vi "Emballage_BDD_bdd_config_emb_Verif.vi"(8 "Error in":errorcluster caption="Error in (no error)", 11 "tableau_config":string[](array[string])) -> (0 "Error out":errorcluster)   [LabVIEW 2020]
uses:
  Modules/Fonction Standard/Email/InfoEmail.ctl
  Modules/FS/60_FS_Controles/60_FS_SetGet.ctl
panel:
  in  "Nom_table":string="Emballage"
  out "resulting string":string
  out "deltaTime [ms]":u32
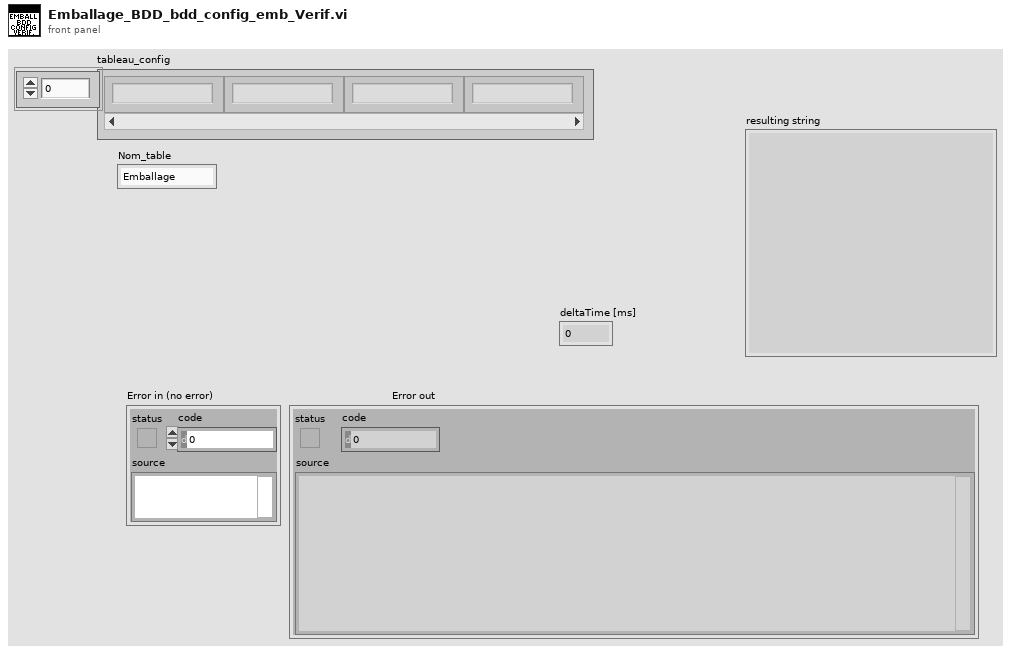
[diagram p1: front panel]
types:
  T1 = typedef "InfoEmail.ctl" = cluster{"Expediteur":string, "Destinataires":string[], "Sujet":string, "Fichier":string, "Message":string}
  T2 = typedef "60_FS_SetGet.ctl" = enum16{"set", "get"}
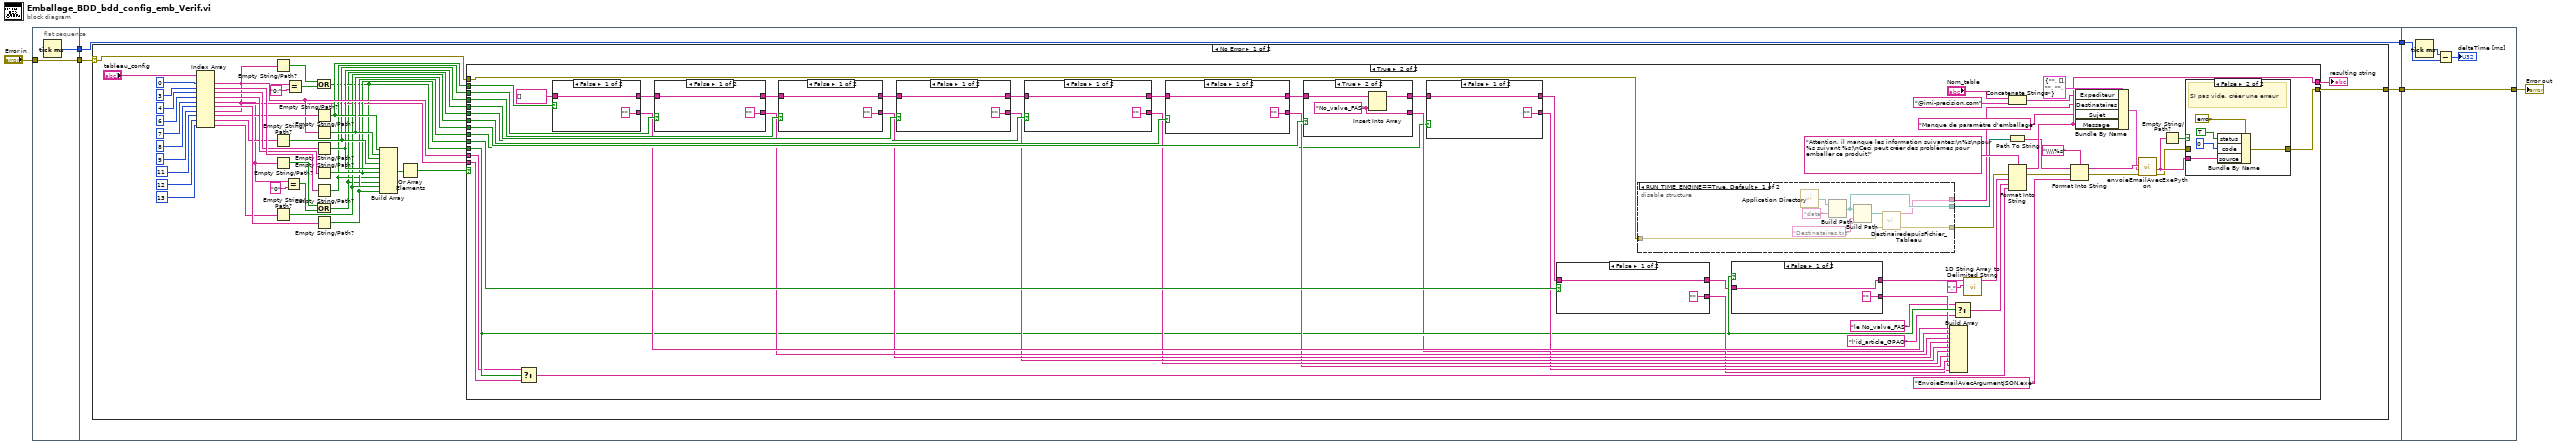
[diagram p0: block diagram]
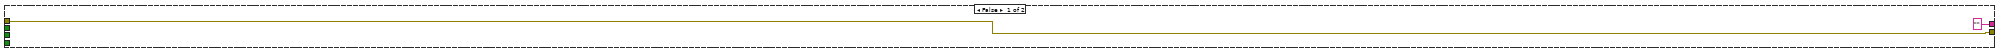
[diagram p2: hidden frame]
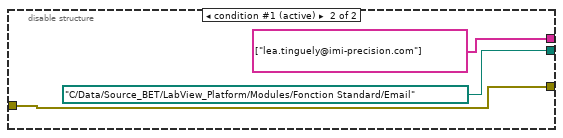
[diagram p3: hidden frame]
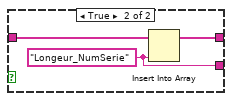
[diagram p5: hidden frame]
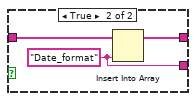
[diagram p6: hidden frame]
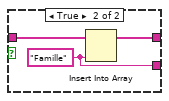
[diagram p7: hidden frame]
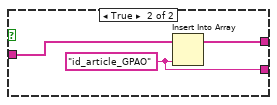
[diagram p8: hidden frame]
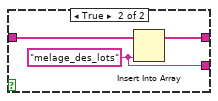
[diagram p9: hidden frame]
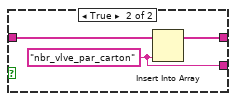
[diagram p10: hidden frame]
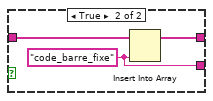
[diagram p11: hidden frame]
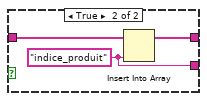
[diagram p12: hidden frame]
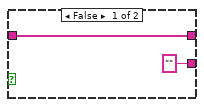
[diagram p13: hidden frame]
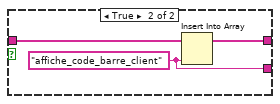
[diagram p14: hidden frame]
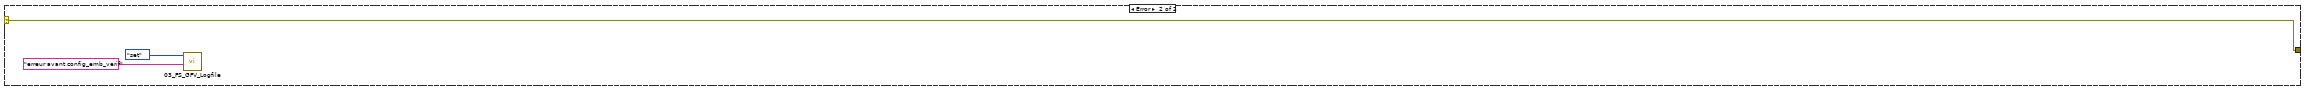
[diagram p15: hidden frame]
diagram:
  n1 = flat-sequence {
    tunnel: "Error in" -> [w8]
    tunnel: [w8] -> w3
    tunnel: [w7] -> w2
    tunnel: [w10] -> w4
    tunnel: w3 -> [w11]
    tunnel: w2 -> [w9]
    tunnel: [w9] -> w1
    tunnel: [w190] -> w5
    tunnel: w4 -> [w190]
    tunnel: w1 -> [w188]
    frame #0 {
      n2 = Tick Count (ms)() -> (millisecond timer value=w7:u32)
    }
    frame #1 {
      n3 = case shown="No Error" w11 {
        selector: w11 -> [w33 w186]
        tunnel: [w34 w186] -> w10
        frame No Error {
          n4 = Index Array(array="tableau_config", index #1=0 ("index"), index #2=3 ("index"), index #3=4 ("index"), index #4=6 ("index"), index #5=7 ("index"), index #6=8 ("index"), index #7=9 ("index"), index #8=11 ("index"), index #9=12 ("index"), index #10=13 ("index")) -> (element #1=w35:string, element #2=w42:string, element #3=w41:string, element #4=w40:string, element #5=w15:string, element #6=w39:string, element #7=w20:string, element #8=w38:string, element #9=w37:string, element #10=w36:string)
          n5 = Empty String/Path?(string/path=w20) -> (empty?=w23:bool)
          n6 = Empty String/Path?(string/path=w37) -> (empty?=w29:bool)
          n7 = Empty String/Path?(string/path=w15) -> (empty?=w13:bool)
          n8 = Empty String/Path?(string/path=w36) -> (empty?=w25:bool)
          n9 = Equal?(x=w15, y="0") -> (x = y?=w12:bool)
          n10 = Equal?(x=w20, y="0;") -> (x = y?=w17:bool)
          n11 = Or(x=w23, y=w17) -> (x .or. y?=w18:bool)
          n12 = Empty String/Path?(string/path=w38) -> (empty?=w30:bool)
          n13 = Empty String/Path?(string/path=w35) -> (empty?=w31:bool)
          n14 = Empty String/Path?(string/path=w41) -> (empty?=w28:bool)
          n15 = Empty String/Path?(string/path=w40) -> (empty?=w27:bool)
          n16 = Empty String/Path?(string/path=w42) -> (empty?=w21:bool)
          n17 = Or(x=w13, y=w12) -> (x .or. y?=w14:bool)
          n18 = Empty String/Path?(string/path=w39) -> (empty?=w24:bool)
          n19 = Build Array(w30, w31, w18, w29, w28, w27, w21, w14, w25, w24) -> (w22:bool[])
          n20 = Or Array Elements(Boolean array=w22) -> (logical OR=w26:bool)
          n21 = case shown="True" w26 {
            tunnel: w31 -> [_ w116]
            tunnel: w21 -> [_ w115]
            tunnel: w28 -> [_ w114]
            tunnel: w27 -> [_ w113]
            tunnel: w14 -> [_ w112]
            tunnel: w24 -> [_ w90]
            tunnel: w30 -> [_ w111]
            tunnel: w29 -> [_ w110]
            tunnel: w25 -> [_ w109]
            tunnel: w18 -> [_ w95]
            tunnel: w35 -> [_ w93]
            tunnel: w20 -> [_ w91]
            tunnel: [w54 w86] -> w34
            tunnel: w33 -> [w54 w58]
            tunnel: ["" w79] -> w32
            frame False {
            }
            frame True {
              n22 = Select(t=w93, s=w95, f=w91) -> (s? t:f=w96:string)
              n23 = case shown="False" w111 {
                tunnel: ["" w147] -> w107
                tunnel: string[] [] ("appended array") -> [w144 w148]
                tunnel: [w144 w146] -> w73
                frame False {
                }
                frame True {
                  w147 = "Famille"
                  n24 = Insert Into Array(array=w148, new element=w147) -> (w146:string[])  [unwired: 1 in]
                }
              }
              n25 = case shown="False" w115 {
                tunnel: ["" w172] -> w106
                tunnel: w73 -> [w169 w173]
                tunnel: [w169 w171] -> w64
                frame False {
                }
                frame True {
                  w172 = "indice_produit"
                  n26 = Insert Into Array(array=w173, new element=w172) -> (w171:string[])  [unwired: 1 in]
                }
              }
              n27 = case shown="False" w110 {
                tunnel: ["" w143] -> w105
                tunnel: [w139 w142] -> w65
                tunnel: w64 -> [w139 w141]
                frame False {
                }
                frame True {
                  w143 = "Date_format"
                  n28 = Insert Into Array(array=w141, new element=w143) -> (w142:string[])  [unwired: 1 in]
                }
              }
              n29 = case shown="False" w114 {
                tunnel: ["" w168] -> w104
                tunnel: [w164 w167] -> w66
                tunnel: w65 -> [w164 w166]
                frame False {
                }
                frame True {
                  w168 = "code_barre_fixe"
                  n30 = Insert Into Array(array=w166, new element=w168) -> (w167:string[])  [unwired: 1 in]
                }
              }
              n31 = case shown="False" w112 {
                tunnel: ["" w163] -> w103
                tunnel: [w159 w162] -> w67
                tunnel: w66 -> [w159 w161]
                frame False {
                }
                frame True {
                  w163 = "nbr_vlve_par_carton"
                  n32 = Insert Into Array(array=w161, new element=w163) -> (w162:string[])  [unwired: 1 in]
                }
              }
              n33 = case shown="False" w109 {
                tunnel: ["" w138] -> w102
                tunnel: [w134 w137] -> w68
                tunnel: w67 -> [w134 w136]
                frame False {
                }
                frame True {
                  w138 = "Longeur_NumSerie"
                  n34 = Insert Into Array(array=w136, new element=w138) -> (w137:string[])  [unwired: 1 in]
                }
              }
              n35 = case shown="True" w116 {
                tunnel: ["" w178] -> w94
                tunnel: [w174 w177] -> w69
                tunnel: w68 -> [w174 w176]
                frame False {
                }
                frame True {
                  w178 = "No_valve_FAS"
                  n36 = Insert Into Array(array=w176, new element=w178) -> (w177:string[])  [unwired: 1 in]
                }
              }
              n37 = case shown="False" w90 {
                tunnel: ["" w158] -> w101
                tunnel: [w154 w157] -> w70
                tunnel: w69 -> [w154 w156]
                frame False {
                }
                frame True {
                  w158 = "melage_des_lots"
                  n38 = Insert Into Array(array=w156, new element=w158) -> (w157:string[])  [unwired: 1 in]
                }
              }
              n39 = case shown="False" w113 {
                tunnel: ["" w183] -> w100
                tunnel: [w179 w182] -> w72
                tunnel: w70 -> [w179 w181]
                frame False {
                }
                frame True {
                  w183 = "affiche_code_barre_client"
                  n40 = Insert Into Array(array=w181, new element=w183) -> (w182:string[])  [unwired: 1 in]
                }
              }
              n41 = disable-structure shown="RUN_TIME_ENGINE==True, Default" {
                disable-tunnel: [w120 path "C:/Data/Source_BET/LabView_Platform/Modules/Fonction Standard/Email" ("appended path")] -> w60
                disable-tunnel: w58 -> [w119 w126]
                disable-tunnel: [w118 w126] -> w57
                disable-tunnel: [w117 string[] ["lea.tinguely@imi-precision.com"]] -> w61
                frame condition #0 {
                  n42 = call <vilib>:"Application Directory.vi"() -> ("Application Directory"=w124:path)
                  n43 = Build Path(base path=w124, name or relative path="data" ("nom ou chemin relatif")) -> (appended path=w120:path)
                  n44 = Build Path(base path=w120, name or relative path="Destinataires.txt" ("nom ou chemin relatif")) -> (appended path=w122:path)
                  n45 = call "DestinairedepuisFichier_Tableau.vi"("entrée d'erreur"=w119, "Chemin"=w122) -> ("sortie d'erreur"=w118:errorcluster, "tableau"=w117:string[])  [unwired: 8 in]
                }
                frame condition #1 (active) {
                }
              }
              n46 = case shown="False" w95 {
                tunnel: ["" w153] -> w92
                tunnel: w72 -> [w149 w152]
                tunnel: [w149 w151] -> w71
                frame False {
                }
                frame True {
                  w153 = "id_article_GPAO"
                  n47 = Insert Into Array(array=w152, new element=w153) -> (w151:string[])  [unwired: 1 in]
                }
              }
              n48 = Build Array(w107, w94, w106, w105, w104, w103, w102, w101, w92, w100) -> ()  [unwired: 1 out]
              n49 = Select(t="le No_valve_FAS", s=w95, f="l'id_article_GPAO") -> (s? t:f=w97:string)
              n50 = call <vilib>:"1D String Array to Delimited String.vi"("delimiter"=",", "string array"=w71) -> ("delimited string"=w98:string)  [unwired: 9 in]
              n51 = Concatenate Strings("Nom_table", "@imi-precision.com" ("chaîne")) -> (w75:string)
              n52 = Path To String(path=w60) -> (string=w59:string)
              n53 = Format Into String(format string="Attention, il manque les information suivantes:\n%s\npour %s suivant %s!\nCeci peut créer des problèmes pour emballer ce produit!", error in=w57, w98, w97, w96) -> (resulting string=w79:string, error out=w83:errorcluster)  [unwired: 1 in]
              n54 = Format Into String(format string="\\\\%s" ("chaîne de format"), initial string=w59, error in=w83, "EnvoieEmailAvecArgumentJSON.exe" ("entrée 1")) -> (resulting string=w82:string, error out=w56:errorcluster)
              n55 = Bundle By Name(cluster=T1 {"Expediteur"="", "Destinataires"=[], "Sujet"="", "Fichier"="", "Message"=""} ("Infos emails"), "Expediteur"=w75, "Destinataires"=w61, "Sujet"="Manque de paramètre d'emballage", "Message"=w79) -> (w80:T1)
              n56 = call "envoieEmailAvecExePython.vi"("error in (no error)"=w56, "Infos emails"=w80, "command line"=w82) -> ("error out"=w87:errorcluster, "standard error"=w88:string)  [unwired: 5 in, 2 out]
              n57 = Empty String/Path?(string/path=w88) -> (empty?=w89:bool)
              n58 = case shown="False" w89 {
                tunnel: w87 -> [w128 _]
                tunnel: [w128 w130] -> w86
                tunnel: w88 -> [_ w129]
                frame True {
                }
                frame False {
                  # "SI pas vide, créer une erreur"
                  n59 = Bundle By Name(cluster=errorcluster {"status"=FALSE, "code"=0, "source"=""} ("constante d'erreur"), "status"=TRUE, "code"=0, "source"=w129) -> (w130:errorcluster)
                }
              }
            }
          }
          "resulting string" <- w32
        }
        frame Error {
          n60 = call "03_FS_GFV_Logfile.vi"("Chaîne"="erreur avant config_emb_verif", "States"=60_FS_SetGet."set") -> ()  [unwired: 8 in, 2 out]
        }
      }
    }
    frame #2 {
      n61 = Tick Count (ms)() -> (millisecond timer value=w189:u32)
      n62 = Subtract(x=w189, y=w188) -> (x-y=→"deltaTime [ms]":u32)
    }
  }
  "Error out" <- w5
